vi "Get measurement.vi"(6 "wait for reply (T)":bool=TRUE, 8 "error in":errorcluster, 9 "Measurement Type":i32(ring) items=["Frequency", "Mean", "Period", "Pulse Duty", "Peak to Peak", "Cycle RMS", "Minimum", "Maximum", "Rise Time", "Fall Time", "Positive Width", "Negative Width", "Amplitude", "Cycle Mean", "High", "Low", "Negative Duty", "Positive Overshoot", "Negative Overshoot", "Cursor Mean", "Burst Width", "Positive Pulse Count", "Negative Pulse Count", "Rising Edge Count", "Falling Edge Count", "Area", "Cycle Area", "RMS", "Cursor RMS"], 10 "Channel":i32(ring)=1 items=["Channel 1"=1, "Channel 2"=2, "Channel 3"=3, "Channel 4"=4], 11 "Module ID":i32=-1) -> (0 "error out":errorcluster, 1 "timed out?":bool, 3 "Value":dbl)   [LabVIEW 2020, in "TDS1002 Oscilloscope.lvlib"]
doc: "Request to get a single measurement from oscilloscope memory.\n_____\nCreated using DQMH Event Scripter 6.1.0.128."
uses:
  TDS1002 Oscilloscope.lvlib
  Get measurement Argument--cluster.ctl
  Get measurement (Reply Payload)--cluster.ctl
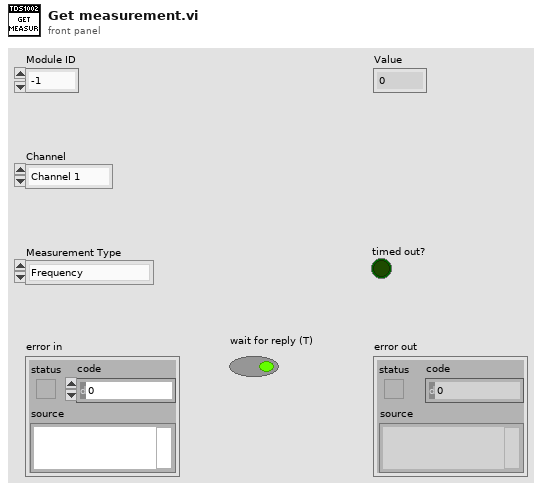
[diagram p1: front panel]
types:
  T1 = typedef "TDS1002 Oscilloscope.lvlib/Get measurement Argument--cluster.ctl" = cluster{"Module ID":i32, "Channel":i32, "Measurement Type":i32, "Wait Notifier":refnum<notifier>, "wait for reply":bool}
  T2 = typedef "TDS1002 Oscilloscope.lvlib/Request Events--cluster.ctl" = cluster{"Stop Module":refnum<user-event>, "Show Panel":refnum<user-event>, "Hide Panel":refnum<user-event>, "Show Diagram":refnum<user-event>, "Get Module Execution Status":refnum<user-event>, "Draw Panel into Subpanel":refnum<user-event>, "Remove Panel from Subpanel":refnum<user-event>, "Connect":refnum<user-event>, "Disconnect":refnum<user-event>, "Configure acquisition":refnum<user-event>, "Configure trigger":refnum<user-event>, "Send software trigger":refnum<user-event>, "Start continuous acquistion":refnum<user-event>, "Stop continuous acquisition":refnum<user-event>, "Get measurement":refnum<user-event>}
  T3 = typedef "TDS1002 Oscilloscope.lvlib/Get measurement (Reply Payload)--cluster.ctl" = cluster{"Value":dbl, "error":errorcluster}
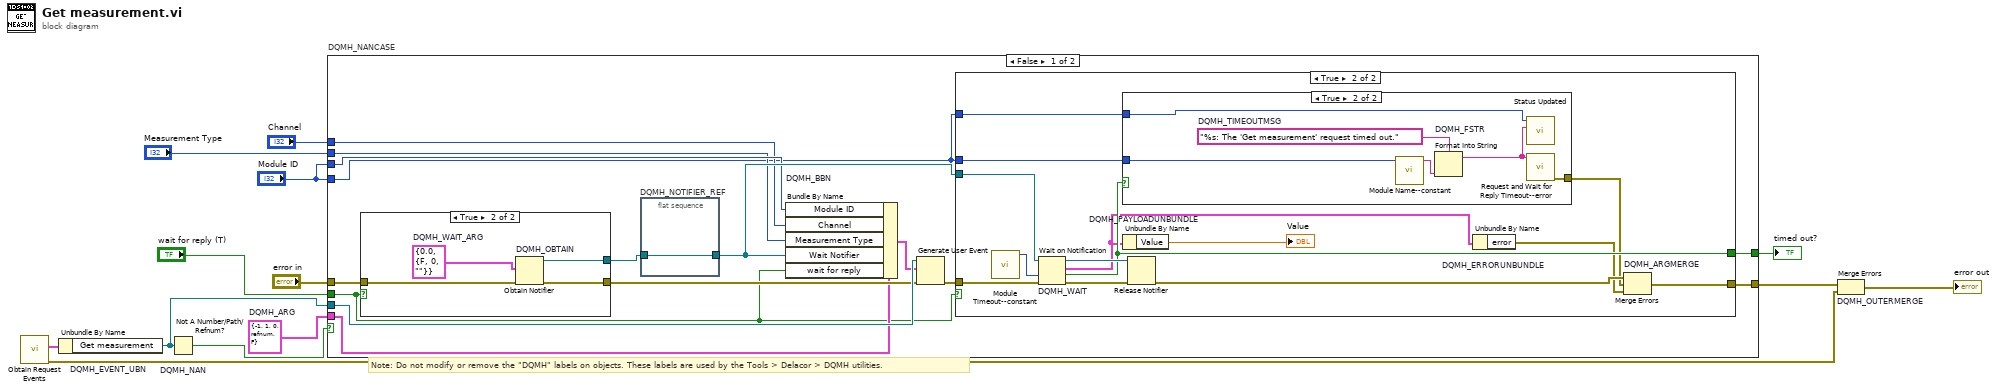
[diagram p0: block diagram]
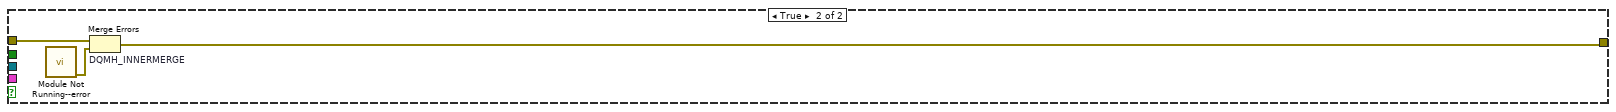
[diagram p5: hidden frame]
diagram:
  w7 = T1 {"Module ID"=-1, "Channel"=1, "Measurement Type"=0, "Wait Notifier"=refnum, "wait for reply"=FALSE}  # DQMH_ARG
  # "Note: Do not modify or remove the \"DQMH\" labels on objects. These labels are used by the Tools > Delacor > DQMH utilities."
  n1 = call "Obtain Request Events.vi"() -> ("error out"=w2:errorcluster, "TDS1002 Oscilloscope Request Events"=w1:T2)  [unwired: 10 in]
  n2 = Unbundle By Name "DQMH_EVENT_UBN"(w1) -> ("Get measurement"=w11:refnum<user-event>)
  n3 = Not A Number/Path/Refnum? "DQMH_NAN"(number/path/refnum=w11) -> (NaN/Path/Refnum?=w10:bool)
  n4 = case "DQMH_NANCASE" shown="False" w10 {
    tunnel: "error in" -> [w28 w58]
    tunnel: w11 -> [w26 _]
    tunnel: [w23 w57] -> w8
    tunnel: [w24 _] -> w9
    tunnel: w7 -> [w19 _]
    tunnel: "Module ID" -> [w18 _]
    tunnel: "Channel" -> [w17 _]
    tunnel: "Measurement Type" -> [w16 _]
    tunnel: "Module ID" -> [w15 _]
    tunnel: "wait for reply (T)" -> [w14 _]
    frame False {
      n5 = case shown="True" w14 {
        tunnel: w28 -> [w51 w55]
        tunnel: [w51 w54] -> w25
        tunnel: [_ w52] -> w21
        frame False {
        }
        frame True {
          w53 = T3 {"Value"=0.0, "error"={"status"=FALSE, "code"=0, "source"=""}}  # DQMH_WAIT_ARG
          n6 = Obtain Notifier "DQMH_OBTAIN"(notification data type=w53, error in (no error)=w55) -> (notifier out=w52:refnum<notifier>, error out=w54:errorcluster)  [unwired: 2 in, 1 out]
        }
      }
      n7 = flat-sequence "DQMH_NOTIFIER_REF" {
        tunnel: w21 -> [w29]
        tunnel: [w29] -> w20
        frame #0 {
        }
      }
      n8 = Bundle By Name "DQMH_BBN"(cluster=w19, "Module ID"=w18, "Channel"=w17, "Measurement Type"=w16, "Wait Notifier"=w20, "wait for reply"=w14) -> (w22:T1)
      n9 = Generate User Event(user event=w26, event data cluster=w22, error in=w25) -> (error out=w27:errorcluster)  [unwired: 1 in, 1 out]
      n10 = case shown="True" w14 {
        tunnel: w27 -> [w30 w44]
        tunnel: w20 -> [_ w43]
        tunnel: [_ w41] -> w24
        tunnel: [w30 w40] -> w23
        tunnel: w15 -> [_ w32]
        tunnel: w15 -> [_ w31]
        frame False {
        }
        frame True {
          n11 = call "Module Timeout--constant.vi"() -> ("Module Timeout"=w34:i32)  [unwired: 11 in]
          n12 = Wait on Notification "DQMH_WAIT"(notifier=w43, timeout in ms (-1)=w34, error in (no error)=w44) -> (notifier out=w42:refnum<notifier>, notification=w35:T3, timed out?=w41:bool, error out=w39:errorcluster)  [unwired: 1 in]
          n13 = case shown="True" w41 {
            tunnel: [_ w48] -> w36
            tunnel: w32 -> [_ w46]
            tunnel: w31 -> [_ w45]
            frame False {
            }
            frame True {
              w50 = "%s: The 'Get measurement' request timed out."  # DQMH_TIMEOUTMSG
              n14 = call "Module Name--constant.vi"("Module ID"=w45) -> ("Module Name"=w47:string)  [unwired: 10 in]
              n15 = Format Into String "DQMH_FSTR"(format string=w50, w47) -> (resulting string=w49:string)  [unwired: 2 in, 1 out]
              n16 = call "Status Updated.vi"("Status"=w49, "Module ID"=w46) -> ()  [unwired: 9 in, 1 out]
              n17 = call "Request and Wait for Reply Timeout--error.vi"("Error Message"=w49) -> ("error out"=w48:errorcluster)  [unwired: 10 in]
            }
          }
          n18 = Unbundle By Name "DQMH_PAYLOADUNBUNDLE"(w35) -> ("Value"=→"Value":dbl)
          n19 = Release Notifier(notifier=w42, error in (no error)=w39) -> (error out=w38:errorcluster)  [unwired: 1 in, 2 out]
          n20 = Unbundle By Name "DQMH_ERRORUNBUNDLE"(w35) -> ("error"=w37:errorcluster)
          n21 = Merge Errors "DQMH_ARGMERGE"(w38, w36, w37) -> (w40:errorcluster)
        }
      }
    }
    frame True {
      n22 = call "Module Not Running--error.vi"() -> ("error out"=w56:errorcluster)  [unwired: 11 in]
      n23 = Merge Errors "DQMH_INNERMERGE"(w58, w56) -> (w57:errorcluster)
    }
  }
  "timed out?" <- w9
  n24 = Merge Errors "DQMH_OUTERMERGE"(w8, w2) -> (→"error out":errorcluster)
